vi "BasicReadWrite.vi"() -> ()   [LabVIEW 2023]
panel:
  out "Thermometer":dbl(slide) scale=0.0..100.0
  out "error out 3":errorcluster
  in  "Voltage 3":u16
  in  "Start Sequence 1":bool
  out "FSM State":string
  in  "VISA Refnum in 2":refnum<visa-resource-name>
  in  "stop 3":bool
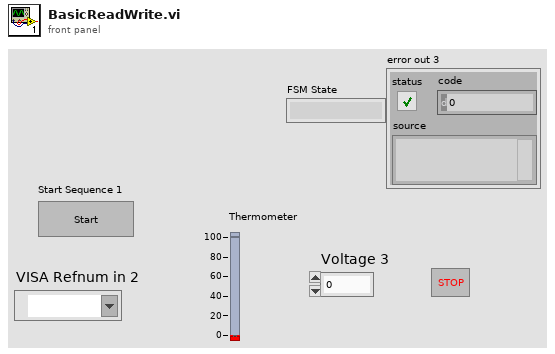
[diagram p1: front panel]
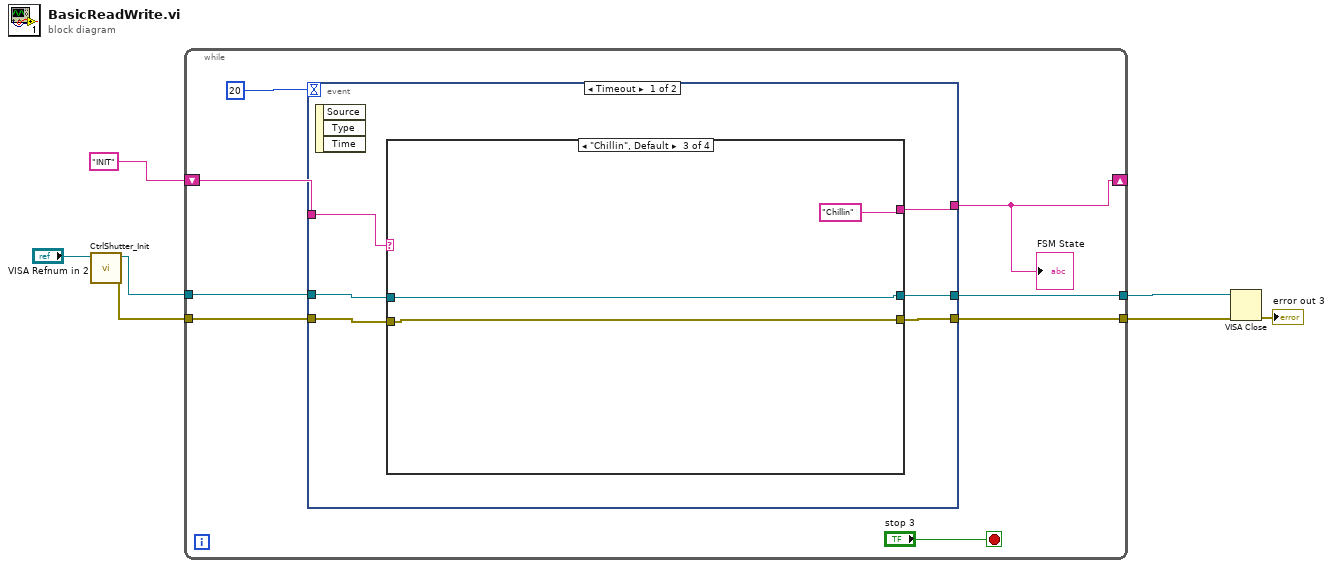
[diagram p0: block diagram]
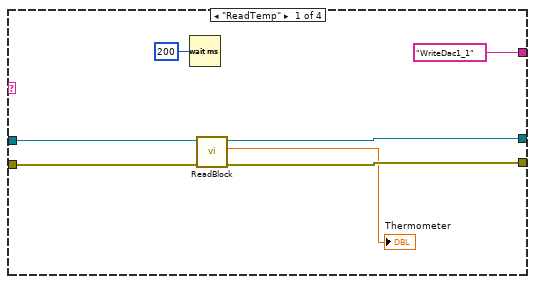
[diagram p2: hidden frame]
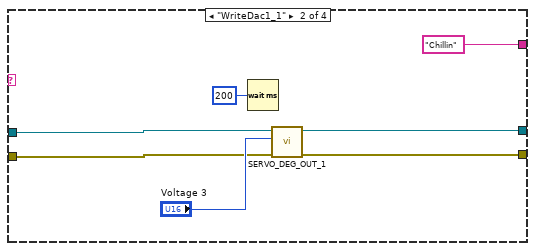
[diagram p3: hidden frame]
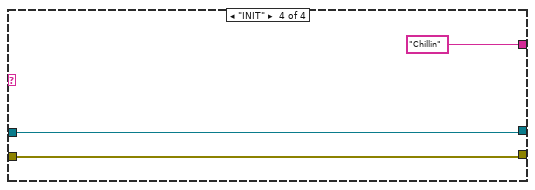
[diagram p4: hidden frame]
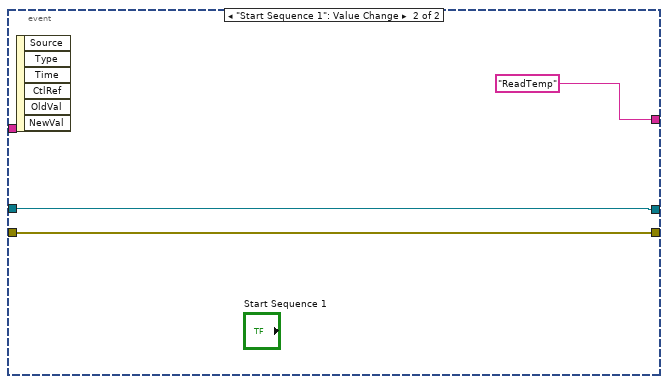
[diagram p5: hidden frame]
diagram:
  n1 = call "CtrlShutter_Init.vi"("VISA Refnum in"="VISA Refnum in 2") -> ("error out"=w4:errorcluster, "VISA Refnum out"=w5:refnum<visa-resource-name>)  [unwired: 8 in, 1 out]
  n2 = while {
    tunnel: w5 -> [w13]
    tunnel: w4 -> [w12]
    tunnel: [w11] -> w2
    tunnel: [w10] -> w1
    shift-right: [w8] -> _
    shift-left: "INIT" ("f") -> [w9]
    stop <- "stop 3" stop-if-true
    n3 = event shown="[0] Timeout" {
      selector: _ -> [_ _]
      dyn-events: _ -> [_ _]
      timeout: 20 -> [_ _]
      tunnel: [w17 "ReadTemp" ("f")] -> w8
      tunnel: w13 -> [w21 w43]
      tunnel: w12 -> [w20 w42]
      tunnel: [w19 w42] -> w11
      tunnel: [w18 w43] -> w10
      tunnel: w9 -> [w16 _]
      event Timeout {
        n4 = event-data() -> ()  [unwired: 1 in, 3 out]
        n5 = case shown="\"Chillin\", Default" w16 {
          tunnel: w21 -> [w27 w33 w36 w39]
          tunnel: w20 -> [w26 w32 w37 w40]
          tunnel: [w25 w31 w37 w40] -> w19
          tunnel: [w24 w29 w36 w39] -> w18
          tunnel: ["WriteDac1_1" "Chillin" "Chillin" "Chillin"] -> w17
          frame "ReadTemp" {
            n6 = Wait (ms)(milliseconds to wait=u32 200) -> ()  [unwired: 1 out]
            n7 = call "ReadBlock.vi"("VISA Refnum in"=w27, "error in (no error)"=w26) -> ("VISA Refnum out"=w24:refnum<visa-resource-name>, "Temperature"=→"Thermometer":dbl, "error out"=w25:errorcluster)  [unwired: 6 in]
          }
          frame "WriteDac1_1" {
            n8 = Wait (ms)(milliseconds to wait=u32 200) -> ()  [unwired: 1 out]
            n9 = call "SERVO_DEG_OUT_1.vi"("VISA Refnum in"=w33, "Voltage"="Voltage 3", "error in (no error)"=w32) -> ("VISA Refnum out"=w29:refnum<visa-resource-name>, "error out"=w31:errorcluster)  [unwired: 5 in, 1 out]
          }
          frame "Chillin", Default {
          }
          frame "INIT" {
          }
        }
      }
      event "Start Sequence 1": Value Change {
        n10 = event-data() -> ()  [unwired: 1 in, 6 out]
      }
    }
    "FSM State" <- w8
  }
  n11 = VISA Close(VISA resource name=w1, error in (no error)=w2) -> (error out=→"error out 3":errorcluster)
